vi "Send experiment info.vi"(8 "error in (no error)":errorcluster, 11 "Tomo in":refnum<class "Tomo.lvclass">) -> (0 "error out":errorcluster, 3 "Tomo out":refnum<class "Tomo.lvclass">)   [LabVIEW 2012, in "Tomo.lvclass"]
uses:
  Tomo.lvclass
  <vilib>/Distrio/Murmex/Murmex/update_cluster.ctl
  Tomo.lvclass/Tomo.ctl
  <vilib>/Distrio/Murmex/Murmex/Murmex.lvclass
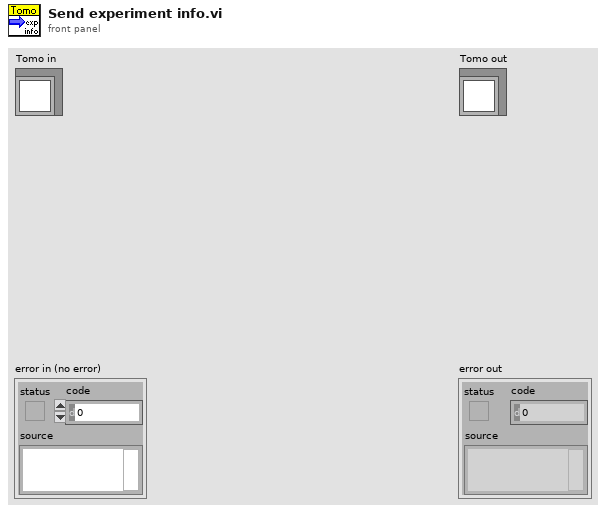
[diagram p1: front panel]
types:
  T1 = typedef "Murmex.lvlib/Murmex.lvclass/update_cluster.ctl" = cluster{"target ID":string, "key chains":string[], "values":variant[]}
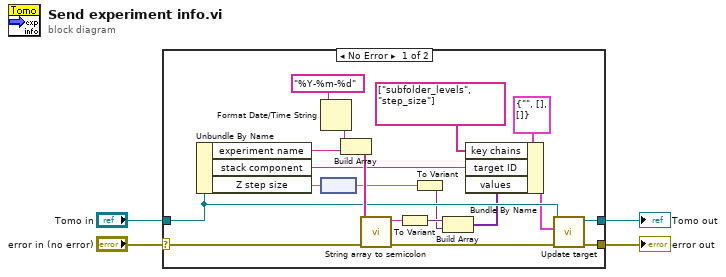
[diagram p0: block diagram]
diagram:
  n1 = case shown="No Error" "error in (no error)" {
    selector: "error in (no error)" -> [w15 w25]
    tunnel: [w18 w25] -> w3
    tunnel: [w16 w24] -> w1
    tunnel: "Tomo in" -> [w17 w24]
    frame No Error {
      n2 = Unbundle By Name(w17) -> ("experiment name"=w21:string, "stack component"=w13:string, "Z step size"=w8:dbl[unit])
      n3 = Format Date/Time String(time format string (%c)="%Y-%m-%d") -> (date/time string=w22:string)  [unwired: 2 in]
      n4 = node(w8) -> (w6:dbl)
      n5 = Build Array(w22, w21) -> (w20:string[])
      n6 = call "String array to semicolon.vi"("error in"=w15, "String array"=w20) -> ("error out"=w14:errorcluster, "Semicolon string"=w7:string)  [unwired: 8 in]
      n7 = To Variant(anything=w7) -> (Variant=w12:variant)
      n8 = To Variant(anything=w6) -> (Variant=w5:variant)
      n9 = Build Array(w12, w5) -> (w11:variant[])
      n10 = Bundle By Name(cluster=T1 {"target ID"="", "key chains"=[], "values"=[]} ("update cluster"), "key chains"=string[] ["subfolder_levels", "step_size"], "target ID"=w13, "values"=w11) -> (w10:T1)
      n11 = call <vilib>:"Update target.vi"("error in (no error)"=w14, "update cluster"=w10, "MurmexBase in"=w17) -> ("error out"=w18:errorcluster, "MurmexBase out"=w16:refnum<class "Tomo.lvclass">)  [unwired: 7 in]
    }
    frame Error {
    }
  }
  "error out" <- w3
  "Tomo out" <- w1
